vi "Configure Sequence (User Defined).vi"(0 "VISA resource name":refnum<visa-resource-name>, 1 "Channel Name (1)":string="1", 3 "User Defined Sequence Beginning Step":bool[](array[boolean]), 4 "Waveform Type (1: Voltage)":i32(ring)=1 items=["Voltage"=1, "Current"=0], 5 "error in (no error)":errorcluster {"code" format="%.0x"}, 6 "User Defined Sequence Level":dbl[](array[numeric]) format="%^.3e", 7 "User Defined Sequence Dwell Time":dbl[](array[numeric]) format="%^.3e", 12 "Sequence Step Number (0)":i32) -> (14 "VISA resource name out":refnum<visa-resource-name>, 19 "error out":errorcluster {"code" format="%.0x"})   [LabVIEW 2014, in "Agilent N6700 Series.lvlib"]
doc: "Configures the user defined sequence.\n\n<b>Note:</b>\nThis VI only applies to the N6705B and N6705C DC Power Analyzer."
uses:
  Agilent N6700 Series.lvlib
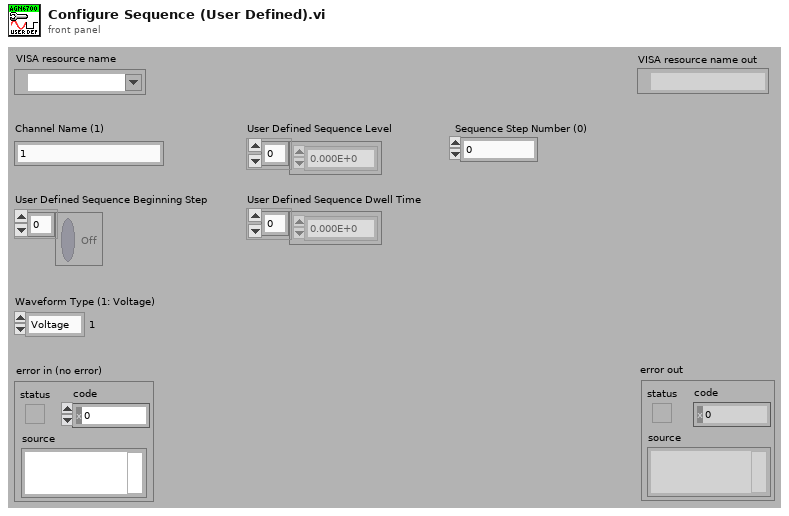
[diagram p1: front panel]
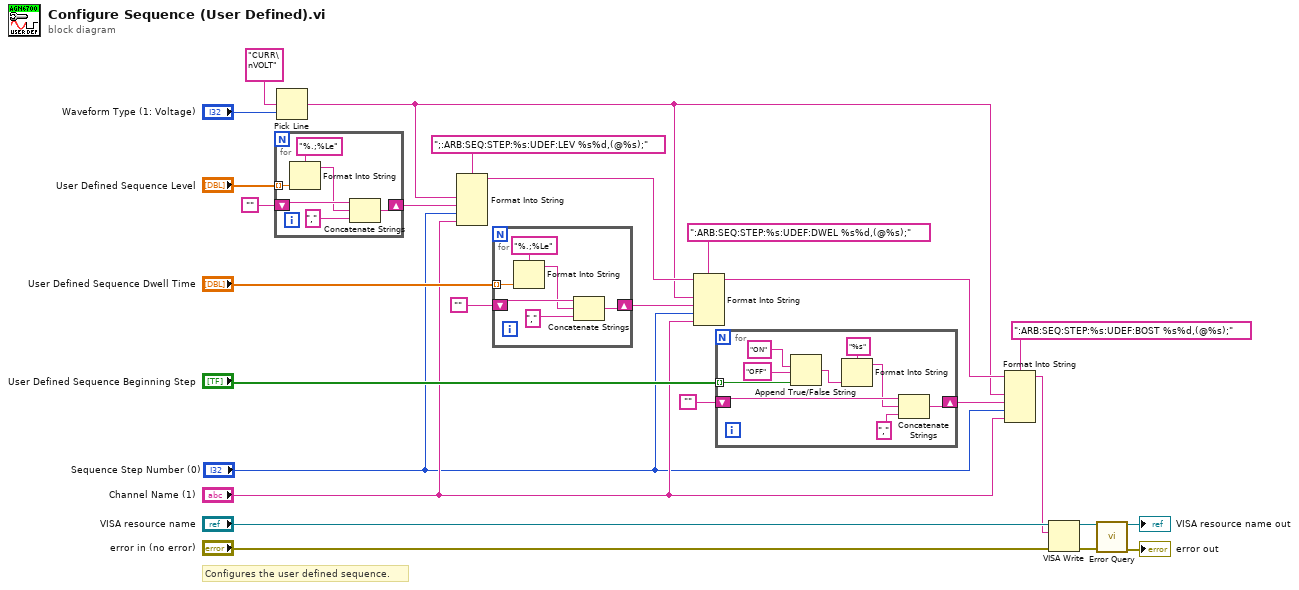
[diagram p0: block diagram]
diagram:
  # "Configures the user defined sequence."
  n1 = for {
    tunnel: "User Defined Sequence Level" -> [w28] mode=indexing
    shift-right: [w32] -> w13
    shift-left: "" ("Empty String Constant") -> [w31]
    n2 = Format Into String(format string="%.;%Le", w28) -> (resulting string=w27:string)  [unwired: 2 in, 1 out]
    n3 = Concatenate Strings(w31, w27, ",") -> (w32:string)
  }
  n4 = Pick Line(multi-line string="CURR\nVOLT", line index="Waveform Type (1: Voltage)") -> (output string=w3:string)  [unwired: 1 in]
  n5 = Format Into String(format string=";:ARB:SEQ:STEP:%s:UDEF:LEV %s%d,(@%s);", w3, w13, "Sequence Step Number (0)", "Channel Name (1)") -> (resulting string=w7:string)  [unwired: 2 in, 1 out]
  n6 = for {
    tunnel: "User Defined Sequence Dwell Time" -> [w34] mode=indexing
    shift-right: [w38] -> w11
    shift-left: "" ("Empty String Constant") -> [w37]
    n7 = Format Into String(format string="%.;%Le", w34) -> (resulting string=w33:string)  [unwired: 2 in, 1 out]
    n8 = Concatenate Strings(w37, w33, ",") -> (w38:string)
  }
  n9 = Format Into String(format string=":ARB:SEQ:STEP:%s:UDEF:DWEL %s%d,(@%s);", initial string=w7, w3, w11, "Sequence Step Number (0)", "Channel Name (1)") -> (resulting string=w4:string)  [unwired: 1 in, 1 out]
  n10 = for {
    tunnel: "User Defined Sequence Beginning Step" -> [w41] mode=indexing
    shift-right: [w47] -> w6
    shift-left: "" ("Empty String Constant") -> [w46]
    n11 = Append True/False String(1:w41, 2:"OFF", 3:"ON") -> (0:w40:string)  [unwired: 1 in]
    n12 = Format Into String(format string="%s", w40) -> (resulting string=w43:string)  [unwired: 2 in, 1 out]
    n13 = Concatenate Strings(w46, w43, ",") -> (w47:string)
  }
  n14 = Format Into String(format string=":ARB:SEQ:STEP:%s:UDEF:BOST %s%d,(@%s);", initial string=w4, w3, w6, "Sequence Step Number (0)", "Channel Name (1)") -> (resulting string=w5:string)  [unwired: 1 in, 1 out]
  n15 = VISA Write(VISA resource name="VISA resource name", write buffer=w5, error in (no error)="error in (no error)") -> (VISA resource name out=w22:refnum<visa-resource-name>, error out=w21:errorcluster)  [unwired: 1 out]
  n16 = call "Error Query.vi"("VISA resource name"=w22, "error in (no error)"=w21) -> ("VISA resource name out"=→"VISA resource name out":refnum<visa-resource-name>, "error out"=→"error out":errorcluster)  [unwired: 10 in, 2 out]
